vi "ALTS-2015 Update Test Selction DO.vi"(8 "error in":errorcluster, 10 "Test Type In":i32, 11 "Station Cluster":T1) -> (0 "error out":errorcluster)   [LabVIEW 2013]
uses:
  Controls/ALTS-2015 Station Cluster.ctl
  SLL DAQ Engine/Software/Source Code/Sub VIs/DAQ Engine/Controls/SLL DE List of Digital Outputs.ctl
  SLL DAQ Engine/Software/Source Code/Sub VIs/DAQ Engine/Controls/SLL DE DO Global Options.ctl
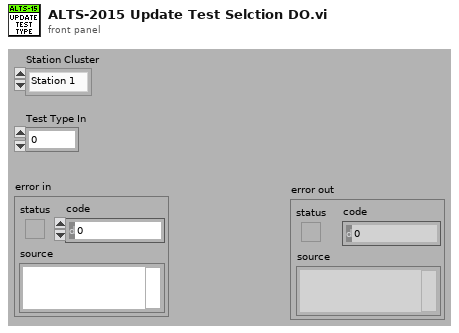
[diagram p1: front panel]
types:
  T1 = typedef "ALTS-2015 Station Cluster.ctl" = enum16{"Station 1", "Station 2", "Station 3", "Station 4"}
  T2 = typedef "SLL DE DO Global Options.ctl" = enum16{"Init", "Write Line", "Write Array", "Write Full Status", "Read Line", "Read Array", "Read Full Status", "Restart DO", "Send to Safe Mode", "Stop DO"}
  T3 = typedef "SLL DE List of Digital Outputs.ctl" = enum16{"STATION1_START TEST", "STATION1_STOP TEST", "STATION1_LIGHT1", "STATION1_LIGHT2", "STATION1_LIGHT3", "STATION1_SELECT_TEST", "STATION2_START TEST", "STATION2_STOP TEST", "STATION2_LIGHT1", "STATION2_LIGHT2", "STATION2_LIGHT3", "STATION2_SELECT_TEST", "STATION3_START TEST", "STATION3_STOP TEST", "STATION3_LIGHT1", "STATION3_LIGHT2", "STATION3_LIGHT3", "STATION3_SELECT_TEST", "STATION4_START TEST", "STATION4_STOP TEST", "STATION4_LIGHT1", "STATION4_LIGHT2", "STATION4_LIGHT3", "STATION4_SELECT_TEST"}
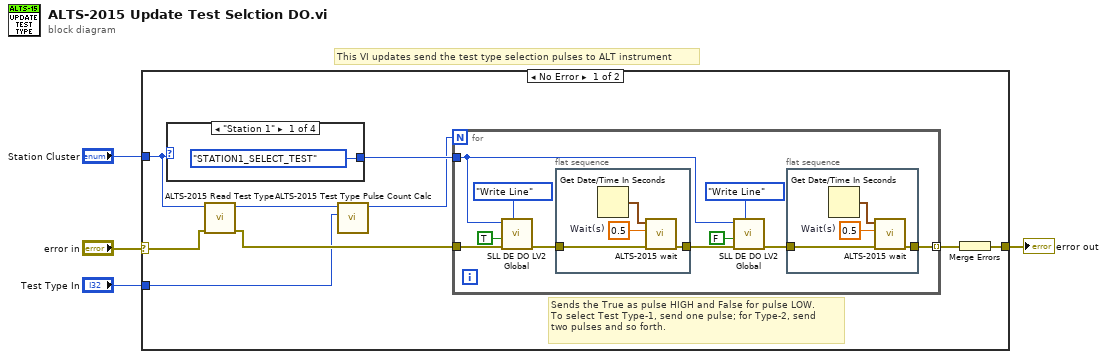
[diagram p0: block diagram]
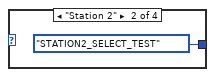
[diagram p2: hidden frame]
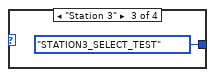
[diagram p3: hidden frame]
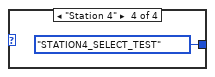
[diagram p4: hidden frame]
diagram:
  # "This VI updates send the test type selection pulses to ALT instrument"
  n1 = case shown="No Error" "error in" {
    selector: "error in" -> [w13 w36]
    tunnel: [w10 w36] -> w4
    tunnel: "Station Cluster" -> [w8 _]
    tunnel: "Test Type In" -> [w5 _]
    frame No Error {
      # "Sends the True as pulse HIGH and False for pulse LOW.\nTo select Test Type-1, send one pulse; for Type-2, send \ntwo pulses and so forth."
      n2 = case shown="\"Station 1\"" w8 {
        tunnel: [SLL_DE_List_of_Digital_Outputs."STATION1_SELECT_TEST" ("DI Channel Name 2") SLL_DE_List_of_Digital_Outputs."STATION2_SELECT_TEST" ("DI Channel Name 2") SLL_DE_List_of_Digital_Outputs."STATION3_SELECT_TEST" ("DI Channel Name 2") SLL_DE_List_of_Digital_Outputs."STATION4_SELECT_TEST" ("DI Channel Name 2")] -> w12
        frame "Station 1" {
        }
        frame "Station 2" {
        }
        frame "Station 3" {
        }
        frame "Station 4" {
        }
      }
      n3 = call "ALTS-2015 Read Test Type.vi"("error in"=w13, "Station Cluster"=w8) -> ("error out"=w9:errorcluster, "Test Type"=w6:i32)  [unwired: 8 in]
      n4 = call "ALTS-2015 Test Type Pulse Count Calc.vi"("Desired Test Type"=w5, "Current Test Type"=w6) -> ("No. of Pulses Required"=w7:i32)  [unwired: 9 in]
      n5 = for {
        N: w7 -> [_]
        tunnel: w9 -> [w22]
        tunnel: w12 -> [w18]
        tunnel: [w14] -> w11 mode=indexing
        n6 = call "SLL DE DO LV2 Global.vi"("DO Option"=SLL_DE_DO_Global_Options."Write Line", "Error In"=w22, "DO State"=TRUE, "DO Channel Name"=w18) -> ("error out"=w20:errorcluster)  [unwired: 4 in, 3 out]
        n7 = flat-sequence {
          tunnel: w20 -> [w29]
          tunnel: [w28] -> w19
          frame #0 {
            w30 = 0.5  # Wait(s)
            n8 = Get Date/Time In Seconds() -> (seconds since 1Jan1904=w31:timestamp)
            n9 = call "ALTS-2015 wait.vi"("error in"=w29, "Wait (s)"=w30, "Start time"=w31) -> ("error out"=w28:errorcluster)  [unwired: 6 in, 2 out]
          }
        }
        n10 = call "SLL DE DO LV2 Global.vi"("DO Option"=SLL_DE_DO_Global_Options."Write Line", "Error In"=w19, "DO State"=FALSE, "DO Channel Name"=w18) -> ("error out"=w15:errorcluster)  [unwired: 4 in, 3 out]
        n11 = flat-sequence {
          tunnel: w15 -> [w25]
          tunnel: [w24] -> w14
          frame #0 {
            w26 = 0.5  # Wait(s)
            n12 = Get Date/Time In Seconds() -> (seconds since 1Jan1904=w27:timestamp)
            n13 = call "ALTS-2015 wait.vi"("error in"=w25, "Wait (s)"=w26, "Start time"=w27) -> ("error out"=w24:errorcluster)  [unwired: 6 in, 2 out]
          }
        }
      }
      n14 = Merge Errors(w11) -> (w10:errorcluster)
    }
    frame Error {
    }
  }
  "error out" <- w4
